vi "Test Print.vi"() -> ()   [LabVIEW 2017]
uses:
  <vilib>/addons/database/Connection.llb/DB Tools Open Connec (String).vi
  <vilib>/Instr/_visa.llb/VISA Configure Serial Port (Instr).vi
  Global/Global 1.vi
  <vilib>/addons/database/NI_Database_API.lvlib
panel:
  in  "DATE CODE 3":string="NB110460ZA210700L27K1234"
  in  "SERIAL NO 3":string="NB110460ZA210700L27K1234"
  in  "print 3":bool
  in  "DATE CODE 2":string="NB110460ZA210700L27K1234"
  in  "SERIAL NO 2":string="NB110460ZA210700L27K1234"
  in  "BBI PART NO":string="NB110460ZA210700L27K1234"
  in  "BRP PART NO":string="NB110460ZA210700L27K1234"
  in  "print 2":bool
  in  "DATE CODE":string="NB110460ZA210700L27K1234"
  in  "BBI PART NO":string="NB110460ZA210700L27K1234"
  in  "SERIAL NO":string="NB110460ZA210700L27K1234"
  in  "BBI DESCRIPTION":string="NB110460ZA210700L27K1234"
  in  "QR DATA":string="NB110460ZA210700L27K1234"
  in  "print 1":bool
  out "result string":string
  out "result PRN":string
  in  "EXIT":bool
  out "error out 2":errorcluster
  in  "error in (no error)":errorcluster
  # "TRECEABILITY"
  # "SATO"
  # "ZEBRA"
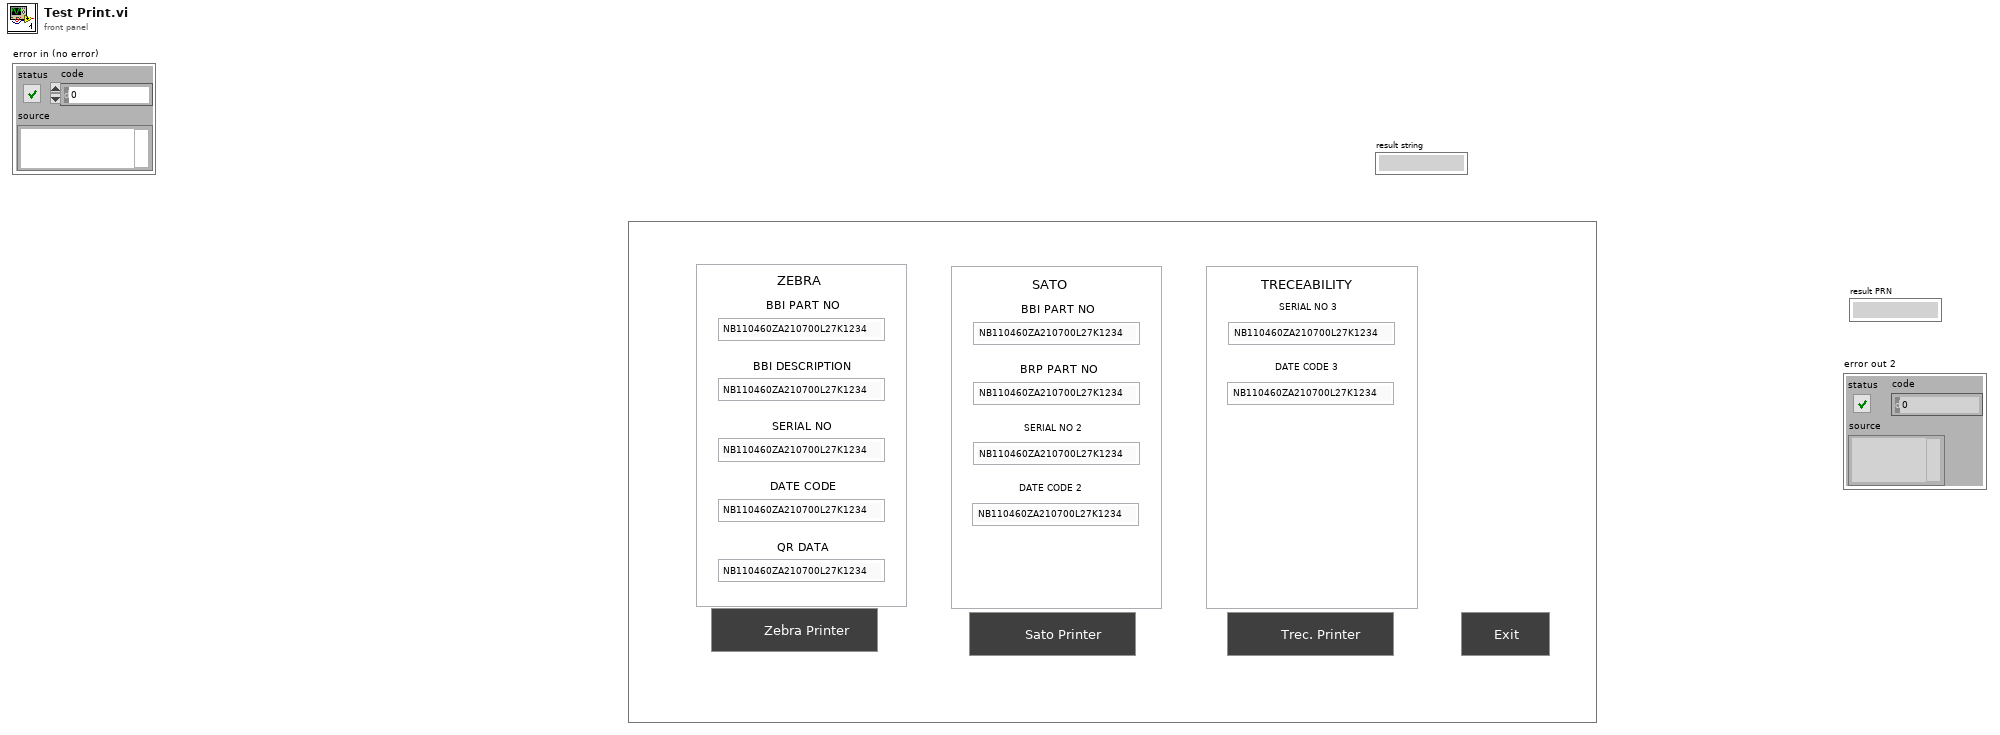
[diagram p1: front panel]
types:
  T1 = typedef "NI_Database_API.lvlib/Conn ObjectReference.ctl" = refnum<k1>
  T2 = enum32{"invalid app kind", "Development System", "Run Time System", "Student Edition", "Embedded LabVIEW", "Evaluation", "Custom"}
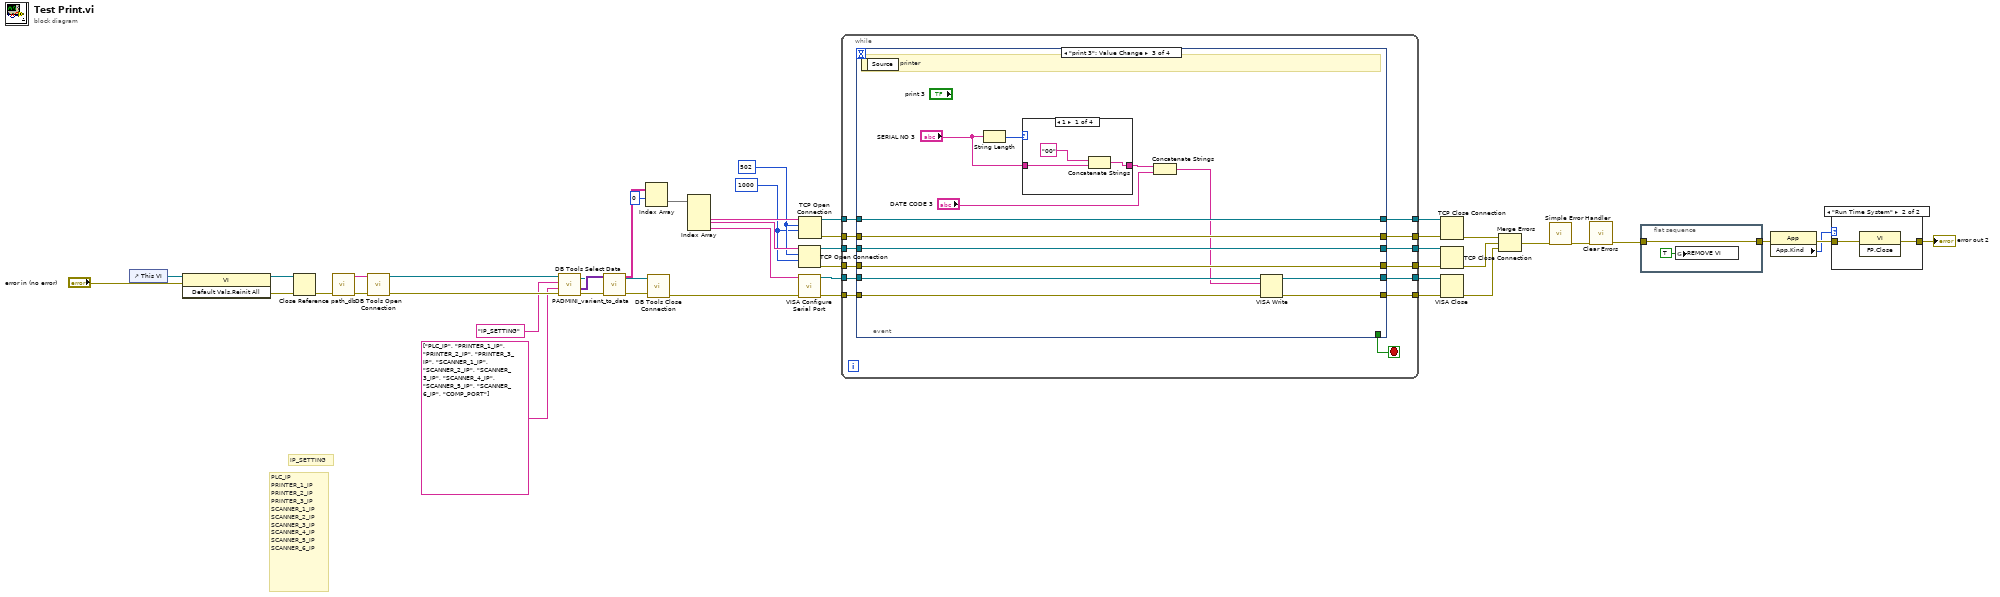
[diagram p0: block diagram]
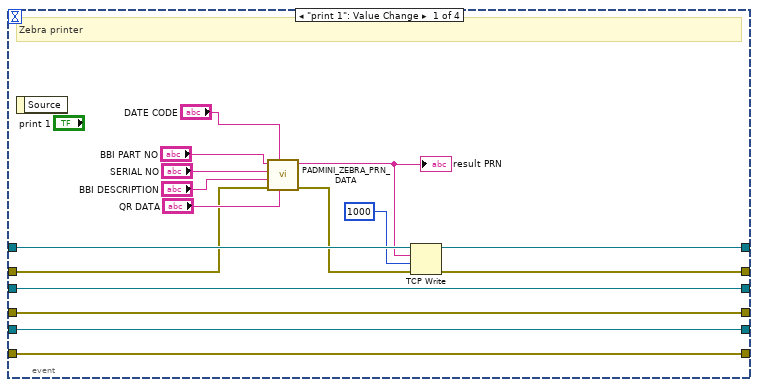
[diagram p2: hidden frame]
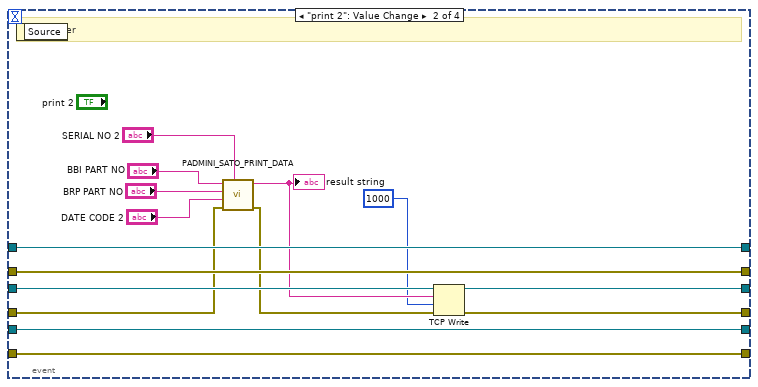
[diagram p3: hidden frame]
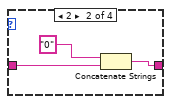
[diagram p4: hidden frame]
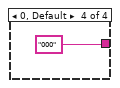
[diagram p6: hidden frame]
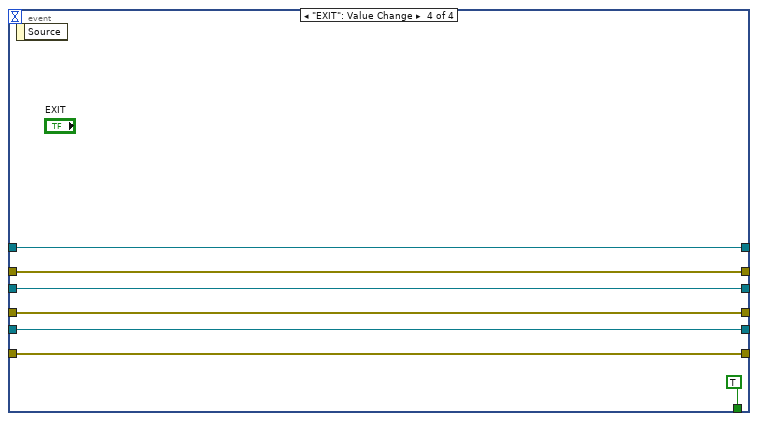
[diagram p7: hidden frame]
diagram:
  w24 = 1000 ("timeout ms (60000)")
  w25 = u16 502 ("remote port or service name")
  # "PLC_IP\nPRINTER_1_IP\nPRINTER_2_IP\nPRINTER_3_IP\nSCANNER_1_IP\nSCANNER_2_IP\nSCANNER_3_IP\nSCANNER_4_IP\nSCANNER_5_IP\nSCANNER_6_IP"
  # "IP_SETTING"
  n1 = control-ref of="This VI"() -> (w46:refnum<vi>)
  n2 = invoke class="VI" method="Default Vals.Reinit All"(reference=w46, error in="error in (no error)") -> (reference out=w44:refnum<vi>, error out=w45:errorcluster)  [unwired: 1 in, 1 out]
  n3 = Close Reference(reference=w44, error in (no error)=w45) -> (error out=w42:errorcluster)
  n4 = call "path_db.vi"("error in"=w42) -> ("error out"=w36:errorcluster, "resulting string"=w41:string)  [unwired: 9 in]
  n5 = call-poly <vilib>:"DB Tools Open Connection.vi"("error in (no error)"=w36, "connection information"=w41) -> ("error out"=w40:errorcluster, "connection reference"=w39:T1)  [unwired: 6 in]
  n6 = call <vilib>:"DB Tools Select Data.vi"("error in (no error)"=w40, "columns"=string[] ["PLC_IP", "PRINTER_1_IP", "PRINTER_2_IP", "PRINTER_3_IP", "SCANNER_1_IP", "SCANNER_2_IP", "SCANNER_3_IP", "SCANNER_4_IP", "SCANNER_5_IP", "SCANNER_6_IP", "COMP_PORT"], "table"="IP_SETTING", "connection reference"=w39) -> ("error out"=w38:errorcluster, "data"=w37:variant[][], "connection reference out"=w32:T1)  [unwired: 2 in]
  n7 = call "PADMINI_varient_to_data.vi"("error in (no error)"=w38, "data"=w37) -> ("error out"=w33:errorcluster, "Array"=w31:string[][])  [unwired: 8 in]
  n8 = Index Array(array=w31, index (row)=0) -> (element=w29:string[])  [unwired: 1 in]
  n9 = call <vilib>:"DB Tools Close Connection.vi"("error in (no error)"=w33, "connection reference"=w32) -> ("error out"=w17:errorcluster)  [unwired: 5 in]
  n10 = Index Array(array=w29) -> (element #2=w28:string, element #3=w27:string, element #4=w26:string)  [unwired: 4 in, 1 out]
  n11 = TCP Open Connection(address=w27, remote port or service name=w25, timeout ms (60000)=w24) -> (connection ID=w21:refnum<k5>, error out=w20:errorcluster)  [unwired: 2 in]
  n12 = call-poly "VISA Configure Serial Port"("VISA resource name"=w26, "error in (no error)"=w17) -> ("VISA resource name out"=w19:refnum<visa-resource-name>, "error out"=w18:errorcluster)  [unwired: 12 in]
  n13 = TCP Open Connection(address=w28, remote port or service name=w25, timeout ms (60000)=w24) -> (connection ID=w23:refnum<k5>, error out=w22:errorcluster)  [unwired: 2 in]
  n14 = while {
    tunnel: w23 -> [w59]
    tunnel: w22 -> [w58]
    tunnel: w21 -> [w57]
    tunnel: w20 -> [w56]
    tunnel: w19 -> [w55]
    tunnel: w18 -> [w54]
    tunnel: [w53] -> w16
    tunnel: [w52] -> w15
    tunnel: [w51] -> w14
    tunnel: [w50] -> w13
    tunnel: [w49] -> w12
    tunnel: [w48] -> w11
    stop <- w47 stop-if-true
    n15 = event shown="[2] \"print 3\": Value Change" {
      selector: _ -> [_ _ _ _]
      dyn-events: _ -> [_ _ _ _]
      timeout: _ -> [_ _ _ _]
      tunnel: w59 -> [w75 w87 w100 w112]
      tunnel: w58 -> [w64 w86 w99 w113]
      tunnel: w57 -> [w72 w90 w98 w114]
      tunnel: w56 -> [w71 w80 w97 w115]
      tunnel: w55 -> [w70 w85 w92 w116]
      tunnel: w54 -> [w69 w84 w103 w117]
      tunnel: [w72 w89 w98 w114] -> w53
      tunnel: [w71 w88 w97 w115] -> w52
      tunnel: [w70 w85 w102 w116] -> w51
      tunnel: [w69 w84 w101 w117] -> w50
      tunnel: [w74 w87 w100 w112] -> w49
      tunnel: [w73 w86 w99 w113] -> w48
      tunnel: [_ _ _ TRUE] -> w47
      event "print 1": Value Change {
        # "Zebra printer"
        n16 = event-data() -> ()  [unwired: 1 in, 1 out]
        n17 = call "PADMINI_ZEBRA_PRN_DATA.vi"("QR DATA"="QR DATA", "DATECODE"="DATE CODE", "error in (no error)"=w64, "BBI DESCRIPTION"="BBI DESCRIPTION", "SERIALNO"="SERIAL NO", "BBI PART NO"="BBI PART NO") -> ("error out"=w63:errorcluster, "result PRN"=w62:string)  [unwired: 4 in]
        "result PRN" <- w62
        n18 = TCP Write(connection ID=w75, data in=w62, error in (no error)=w63, 9:1000 ("timeout ms (25000)")) -> (connection ID out=w74:refnum<k5>, error out=w73:errorcluster)  [unwired: 1 out]
      }
      event "print 2": Value Change {
        # "sato printer"
        n19 = event-data() -> ()  [unwired: 1 in, 1 out]
        n20 = call "PADMINI_SATO_PRINT_DATA.vi"("SERIAL NO"="SERIAL NO 2", "error in (no error)"=w80, "DATE CODE"="DATE CODE 2", "BRP PART NO"="BRP PART NO", "BBI PART NO"="BBI PART NO") -> ("error out"=w79:errorcluster, "result string"=w81:string)  [unwired: 4 in, 1 out]
        "result string" <- w81
        n21 = TCP Write(connection ID=w90, data in=w81, error in (no error)=w79, 9:1000 ("timeout ms (25000)")) -> (connection ID out=w89:refnum<k5>, error out=w88:errorcluster)  [unwired: 1 out]
      }
      event "print 3": Value Change {
        # "treceability printer"
        n22 = event-data() -> ()  [unwired: 1 in, 1 out]
        n23 = String Length(string="SERIAL NO 3") -> (length=w96:i32)
        n24 = case shown="1" w96 {
          tunnel: [w104 w107 w110 "000"] -> w95
          tunnel: "SERIAL NO 3" -> [w105 w108 w110 _]
          frame 1 {
            n25 = Concatenate Strings("00", w105) -> (w104:string)
          }
          frame 2 {
            n26 = Concatenate Strings("0", w108) -> (w107:string)
          }
          frame 3 {
          }
          frame 0, Default {
          }
        }
        n27 = Concatenate Strings(w95, "DATE CODE 3") -> (w91:string)
        n28 = VISA Write(VISA resource name=w92, write buffer=w91, error in (no error)=w103) -> (VISA resource name out=w102:refnum<visa-resource-name>, error out=w101:errorcluster)  [unwired: 1 out]
      }
      event "EXIT": Value Change {
        n29 = event-data() -> ()  [unwired: 1 in, 1 out]
      }
    }
  }
  n30 = TCP Close Connection(connection ID=w12, error in (no error)=w11) -> (error out=w10:errorcluster)  [unwired: 1 in, 1 out]
  n31 = TCP Close Connection(connection ID=w16, error in (no error)=w15) -> (error out=w9:errorcluster)  [unwired: 1 in, 1 out]
  n32 = VISA Close(VISA resource name=w14, error in (no error)=w13) -> (error out=w8:errorcluster)
  n33 = Merge Errors(w10, w9, w8) -> (w7:errorcluster)
  n34 = call <vilib>:"Simple Error Handler.vi"("error in (no error)"=w7) -> ("error out"=w6:errorcluster)  [unwired: 4 in, 4 out]
  n35 = call <vilib>:"Clear Errors.vi"("error in (no error)"=w6) -> ("error out"=w1:errorcluster)  [unwired: 5 in, 1 out]
  n36 = flat-sequence {
    tunnel: w1 -> [w120]
    tunnel: [w120] -> w2
    frame #0 {
      n37 = global write "Global 1.vi" "REMOVE VI"(TRUE ("remove_VI")) -> ()
    }
  }
  n38 = property class="App"(error in=w2) -> (error out=w4:errorcluster, "App.Kind"=w3:T2)  [unwired: 1 in, 1 out]
  n39 = case shown="\"Run Time System\"" w3 {
    tunnel: [w121 w123] -> w5
    tunnel: w4 -> [w121 w122]
    frame "Development System", Default {
    }
    frame "Run Time System" {
      n40 = invoke class="VI" method="FP.Close"(error in=w122) -> (error out=w123:errorcluster)  [unwired: 2 in, 2 out]
    }
  }
  "error out 2" <- w5
